vi "Update Value.vi"(6 "Time":dbl, 8 "error in (no error)":errorcluster, 11 "LoggingControl in":refnum<class "LoggingControl.lvclass">) -> (0 "error out":errorcluster, 1 "Update":bool, 2 "Value":variant, 3 "LoggingControl out":refnum<class "LoggingControl.lvclass">)   [LabVIEW 2020, in "VolatusGUIElements.lvlib" / "LoggingControl.lvclass"]
uses:
  LoggingControl.lvclass
  LoggingControl.lvclass/LoggingControl.ctl
  lv-vecto/Vecto/Channel STR/Channel STR.lvclass/Channel STR.ctl
  lv-vecto/Vecto/Group STR/String by Index.vi
  Loop Async.vi
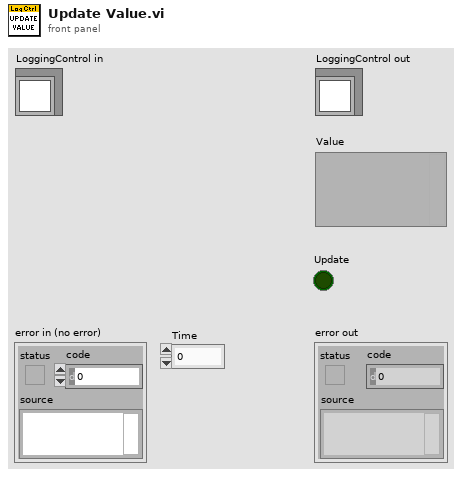
[diagram p1: front panel]
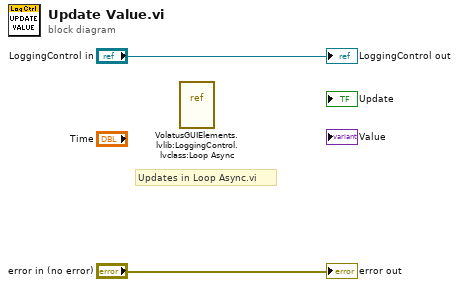
[diagram p0: block diagram]
diagram:
  # "Updates in Loop Async.vi"
  n1 = vi-ref "VolatusGUIElements.lvlib:LoggingControl.lvclass:Loop Async.vi"() -> ()  [unwired: 1 out]
  "error out" <- "error in (no error)"
  "LoggingControl out" <- "LoggingControl in"
